vi "Set parameters.vi"(8 "error in":errorcluster, 11 "DAQ":T1={"Data"={"Live"={"t0"=timestamp(0 s since 1904-01-01), "dt"=1.0, "Y"=[]}, "Accumulated"={"t0"=timestamp(0 s since 1904-01-01), "dt"=1.0, "Y"=[]}, "Averaged"={"t0"=timestamp(0 s since 1904-01-01), "dt"=1.0, "Y"=[]}, "data array"=[], "live time array"=[], "Live (decimated)"={"t0"=timestamp(0 s since 1904-01-01), "dt"=1.0, "Y"=[]}}, "Config"={"Input Config"=0, "Card"=enum."USB-6211", "100% Reflectance Standard (V)"=0.0, "Input Channel"="", "Average number of points"=0.0, "Trigger Level (V)"=0.0, "Rate (Hz)"=0, "End Time (s)"=0.0}, "Indicators"={"Final number of points"=0.0, "Number of samples"=0.0, "dt"=0.0, "Shots"=10, "Shot counter"=10, "Test counter"=10, "Background level (V)"=0.0, "DAQ task"="", "timestamp of data"=timestamp(0 s since 1904-01-01), "Test Type"=enum."A-Test"}} {"Config"."Input Config" items=["default"=-1, "RSE"=10083, "NRSE"=10078, "Differential"=10106, "Pseudodifferential"=12529]}) -> (0 "error out":errorcluster, 3 "DAQ out":T1={"Data"={"Live"={"t0"=timestamp(0 s since 1904-01-01), "dt"=1.0, "Y"=[]}, "Accumulated"={"t0"=timestamp(0 s since 1904-01-01), "dt"=1.0, "Y"=[]}, "Averaged"={"t0"=timestamp(0 s since 1904-01-01), "dt"=1.0, "Y"=[]}, "data array"=[], "live time array"=[], "Live (decimated)"={"t0"=timestamp(0 s since 1904-01-01), "dt"=1.0, "Y"=[]}}, "Config"={"Input Config"=0, "Card"=enum."USB-6211", "100% Reflectance Standard (V)"=0.0, "Input Channel"="", "Average number of points"=0.0, "Trigger Level (V)"=0.0, "Rate (Hz)"=0, "End Time (s)"=0.0}, "Indicators"={"Final number of points"=0.0, "Number of samples"=0.0, "dt"=0.0, "Shots"=10, "Shot counter"=10, "Test counter"=10, "Background level (V)"=0.0, "DAQ task"="", "timestamp of data"=timestamp(0 s since 1904-01-01), "Test Type"=enum."A-Test"}} {"Config"."Input Config" items=["default"=-1, "RSE"=10083, "NRSE"=10078, "Differential"=10106, "Pseudodifferential"=12529]})   [LabVIEW 2017, in "DAQ.lvlib"]
uses:
  DAQ.lvlib
  Controls/Params.ctl
  Controls/DAQ Config.ctl
  Controls/DAQ Indicators.ctl
  System Control/CTLs/Test Type.ctl
  System Control/Main controller.lvlib
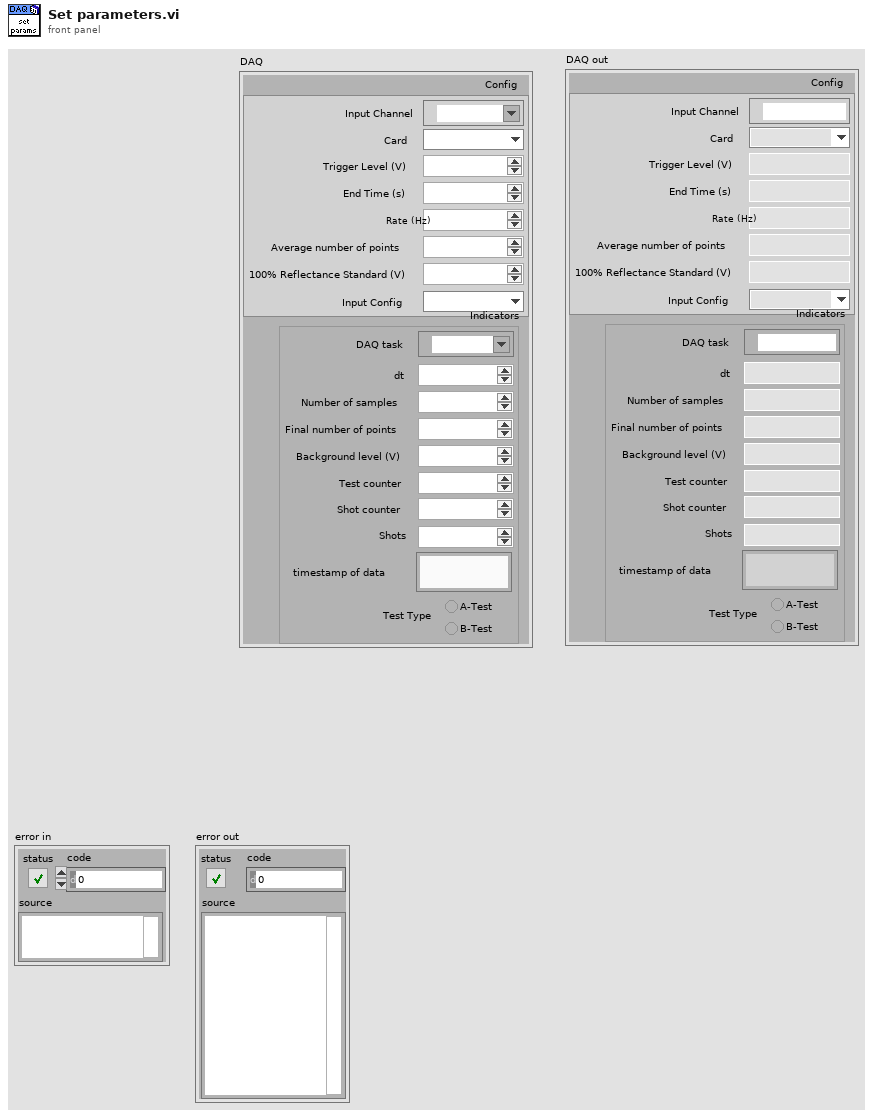
[diagram p1: front panel]
types:
  T1 = typedef "DAQ.lvlib/Params.ctl" = cluster{"Data":cluster{"Live":waveform(dbl), "Accumulated":waveform(dbl), "Averaged":waveform(dbl), "data array":dbl[], "live time array":dbl[], "Live (decimated)":waveform(dbl)}, "Config":T2, "Indicators":T3}
  T2 = typedef "DAQ.lvlib/DAQ Config.ctl" = cluster{"Input Config":i32, "Card":enum16{"USB-6211", "USB-6251", "USB-6361"}, "100% Reflectance Standard (V)":dbl, "Input Channel":tag, "Average number of points":dbl, "Trigger Level (V)":dbl, "Rate (Hz)":i32, "End Time (s)":dbl}
  T3 = typedef "DAQ.lvlib/DAQ Indicators.ctl" = cluster{"Final number of points":dbl, "Number of samples":dbl, "dt":dbl, "Shots":i32, "Shot counter":i32, "Test counter":i32, "Background level (V)":dbl, "DAQ task":refnum<k21>, "timestamp of data":timestamp, "Test Type":T4}
  T4 = typedef "Main controller.lvlib/Test Type.ctl" = enum32{"A-Test", "B-Test"}
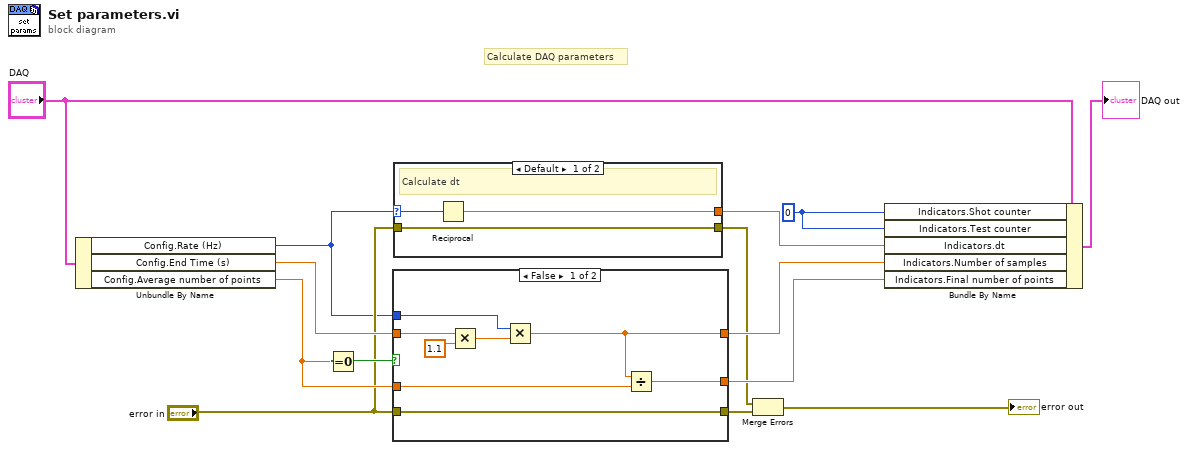
[diagram p0: block diagram]
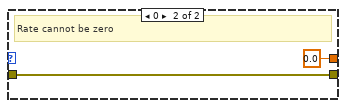
[diagram p2: hidden frame]
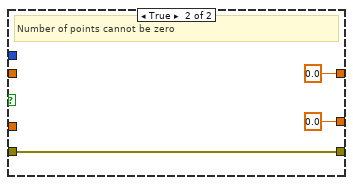
[diagram p3: hidden frame]
diagram:
  w2 = 0 ("Test counter")
  # "Calculate DAQ parameters"
  n1 = Unbundle By Name("DAQ") -> ("Config.Rate (Hz)"=w1:i32, "Config.End Time (s)"=w11:dbl, "Config.Average number of points"=w8:dbl)
  n2 = Equal To 0?(x=w8) -> (x = 0?=w9:bool)
  n3 = case shown="False" w9 {
    tunnel: [w22 0.0] -> w14
    tunnel: [w21 0.0] -> w13
    tunnel: w1 -> [w18 _]
    tunnel: w11 -> [w17 _]
    tunnel: w8 -> [w16 _]
    tunnel: [w15 w23] -> w4
    tunnel: "error in" -> [w15 w23]
    frame False {
      n4 = Multiply(x=w17, y=1.1) -> (x*y=w20:dbl)
      n5 = Multiply(x=w18, y=w20) -> (x*y=w21:dbl)
      n6 = Divide(x=w21, y=w16) -> (x/y=w22:dbl)
    }
    frame True {
      # "Number of points cannot be zero"
    }
  }
  n7 = case shown="Default" w1 {
    selector: w1 -> [w26 _]
    tunnel: [w28 0.0] -> w7
    tunnel: "error in" -> [w27 w29]
    tunnel: [w27 w29] -> w5
    frame Default {
      # "Calculate dt"
      n8 = Reciprocal(x=w26) -> (1/x=w28:dbl)
    }
    frame 0 {
      # "Rate cannot be zero"
    }
  }
  n9 = Merge Errors(w5, w4) -> (→"error out":errorcluster)
  n10 = Bundle By Name(cluster="DAQ", "Indicators.Shot counter"=w2, "Indicators.Test counter"=w2, "Indicators.dt"=w7, "Indicators.Number of samples"=w13, "Indicators.Final number of points"=w14) -> (→"DAQ out":T1)
